vi "DIM_Read Item (Src.SysLab).vi"(8 "error in (no error)":errorcluster, 10 "Sourcer.SysLabel":string, 11 "UI_Actor in":refnum<class "UI_Actor.lvclass">) -> (0 "error out":errorcluster, 1 "Found?":bool, 2 "DIM Item":T1, 3 "UI_Actor out":refnum<class "UI_Actor.lvclass">)   [LabVIEW 2020, in "UI_Actor.lvlib" / "UI_Actor.lvclass"]
uses:
  UI_Actor.lvclass
  ctl_InternalMapItem.ctl
  support/Databox.lvlibp/TypesTools/Config/Config.lvclass
  support/Databox.lvlibp/TypesTools/Data/Data.lvclass
  UI_Actor.lvclass/UI_Actor.ctl
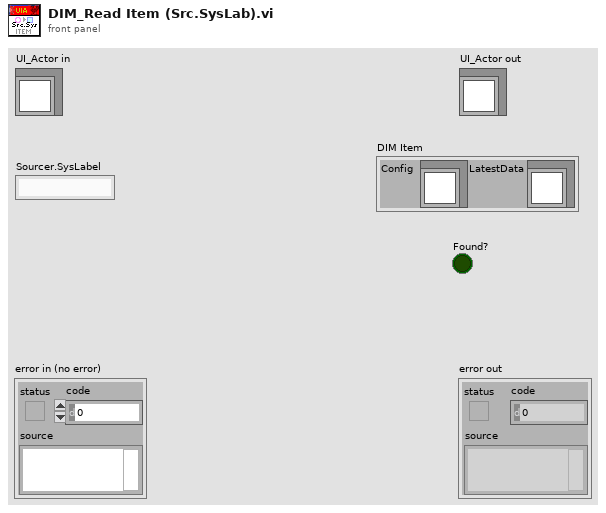
[diagram p1: front panel]
types:
  T1 = typedef "UI_Actor.lvlib/UI_Actor.lvclass/ctl_InternalMapItem.ctl" = cluster{"Config":refnum<class "Config.lvclass">, "LatestData":refnum<class "Data.lvclass">}
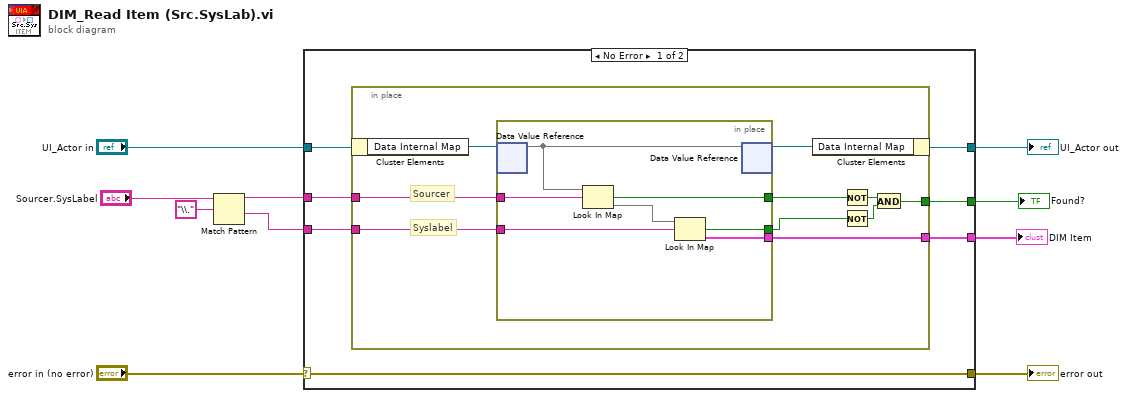
[diagram p0: block diagram]
diagram:
  n1 = Match Pattern(string="Sourcer.SysLabel", regular expression="\\.") -> (before substring=w2:string, after substring=w1:string)  [unwired: 1 in, 2 out]
  n2 = case shown="No Error" "error in (no error)" {
    selector: "error in (no error)" -> [w17 w36]
    tunnel: [w17 w36] -> w9
    tunnel: [w15 w35] -> w7
    tunnel: "UI_Actor in" -> [w16 w35]
    tunnel: w2 -> [w14 _]
    tunnel: [w13 _] -> w6
    tunnel: [w12 _] -> w5
    tunnel: w1 -> [w11 _]
    frame No Error {
      n3 = in-place {
        in-place-border: w14 -> [w25]
        in-place-border: [w24] -> w13
        in-place-border: [w18] -> w12
        in-place-border: w11 -> [w22]
        # "Syslabel"
        # "Sourcer"
        n4 = in-place-cluster #1(w16) -> ("Data Internal Map"=w27:refnum<data-value>)
        n5 = in-place {
          in-place-border: w25 -> [w33]
          in-place-border: [w29] -> w24
          in-place-border: [w32] -> w23
          in-place-border: w22 -> [w30]
          in-place-border: [w28] -> w21
          n6 = in-place-dvr #2(w27) -> (w34:map{string, map{string, T1}})  [unwired: 1 out]
          n7 = Look In Map(map=w34, key=w33) -> (key not found?=w32:bool, value=w31:map{string, T1})  [unwired: 1 in]
          n8 = Look In Map(map=w31, key=w30) -> (key not found?=w28:bool, value=w29:T1)  [unwired: 1 in]
          n9 = in-place-dvr #2(w34) -> (w26:refnum<data-value>)  [unwired: 1 out]
        }
        n10 = in-place-cluster #1("Data Internal Map"=w26) -> (w15:refnum<class "UI_Actor.lvclass">)
        n11 = Not(x=w23) -> (.not. x?=w20:bool)
        n12 = Not(x=w21) -> (.not. x?=w19:bool)
        n13 = And(x=w20, y=w19) -> (x .and. y?=w18:bool)
      }
    }
    frame Error {
    }
  }
  "error out" <- w9
  "UI_Actor out" <- w7
  "DIM Item" <- w6
  "Found?" <- w5
